vi "read available sequences.vi"(8 "error in (no error)":errorcluster, 11 "Simple Sequencer API in":refnum<class "Simple Sequencer API.lvclass">) -> (0 "error out":errorcluster, 2 "available sequences":string[](array[string]), 3 "Simple Sequencer API out":refnum<class "Simple Sequencer API.lvclass">)   [LabVIEW 2014, in "Simple Sequencer API.lvclass"]
doc: "Returns a list of all sequences the sequencer is able to run."
uses:
  Simple Sequencer API.lvclass
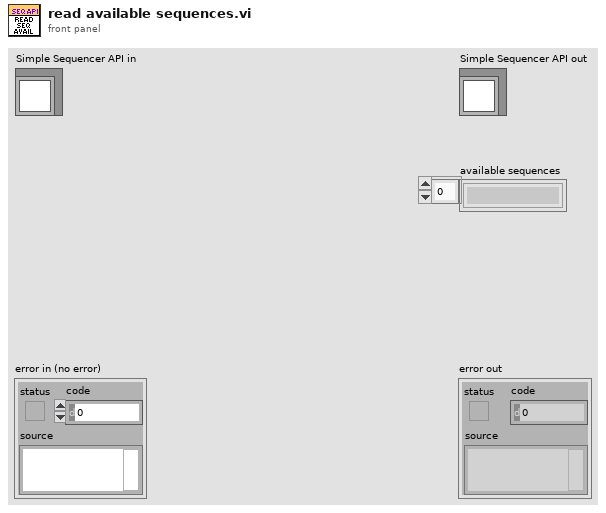
[diagram p1: front panel]
types:
  T1 = typedef "Simple Sequencer TBM configuration.lvclass/sequence definition.ctl" = cluster{"sequence name":string, "action configs":refnum<class "action configuration.lvclass">[]}
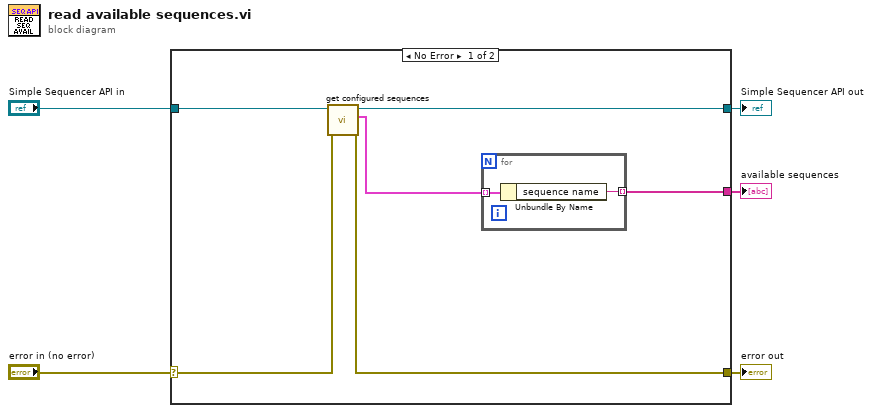
[diagram p0: block diagram]
diagram:
  n1 = case shown="No Error" "error in (no error)" {
    selector: "error in (no error)" -> [w9 w15]
    tunnel: [w8 w15] -> w4
    tunnel: [w6 w14] -> w2
    tunnel: "Simple Sequencer API in" -> [w10 w14]
    tunnel: [w11 _] -> w1
    frame No Error {
      n2 = call "get configured sequences.vi"("error in (no error)"=w9, "Simple Sequencer API in"=w10) -> ("error out"=w8:errorcluster, "sequence definitions"=w7:T1[], "Simple Sequencer API out"=w6:refnum<class "Simple Sequencer API.lvclass">)  [unwired: 7 in]
      n3 = for {
        tunnel: w7 -> [w13] mode=indexing
        tunnel: [w12] -> w11 mode=indexing
        n4 = Unbundle By Name(w13) -> ("sequence name"=w12:string)
      }
    }
    frame Error {
    }
  }
  "error out" <- w4
  "Simple Sequencer API out" <- w2
  "available sequences" <- w1
